vi "QCA.vi"() -> ()   [LabVIEW 2010]
uses:
  QCA Global.vi
panel:
  out "Sweep Done":refnum<k4>
  out "Mode Changed":refnum<k4>
  in  "stop":bool
  in  "Mode":T1(ring)
  out "QCA Message Type":T2(ring)=enum."MonitorDelay="
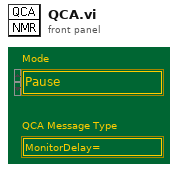
[diagram p1: front panel]
types:
  T1 = enum16{"Pause", "Take Data", "One Point", "NMR Tune", "Monitor"}
  T2 = enum16{"No Message", "Bad Message", "Init", "ChannelFile=", "RF On", "RF Off", "RFFreq=", "RFMod=", "RFPower=", "YaleGain=", "ScanSweeps=", "ScanSteps=", "ScanFreq=", "CalConst=", "MonitorDelay=", "Baseline=", "Baseline", "SaveChans", "Channel=", "Pause", "TakeData", "OnePoint", "NMRTune", "Monitor", "Address=", "Ping=", "Stop"}
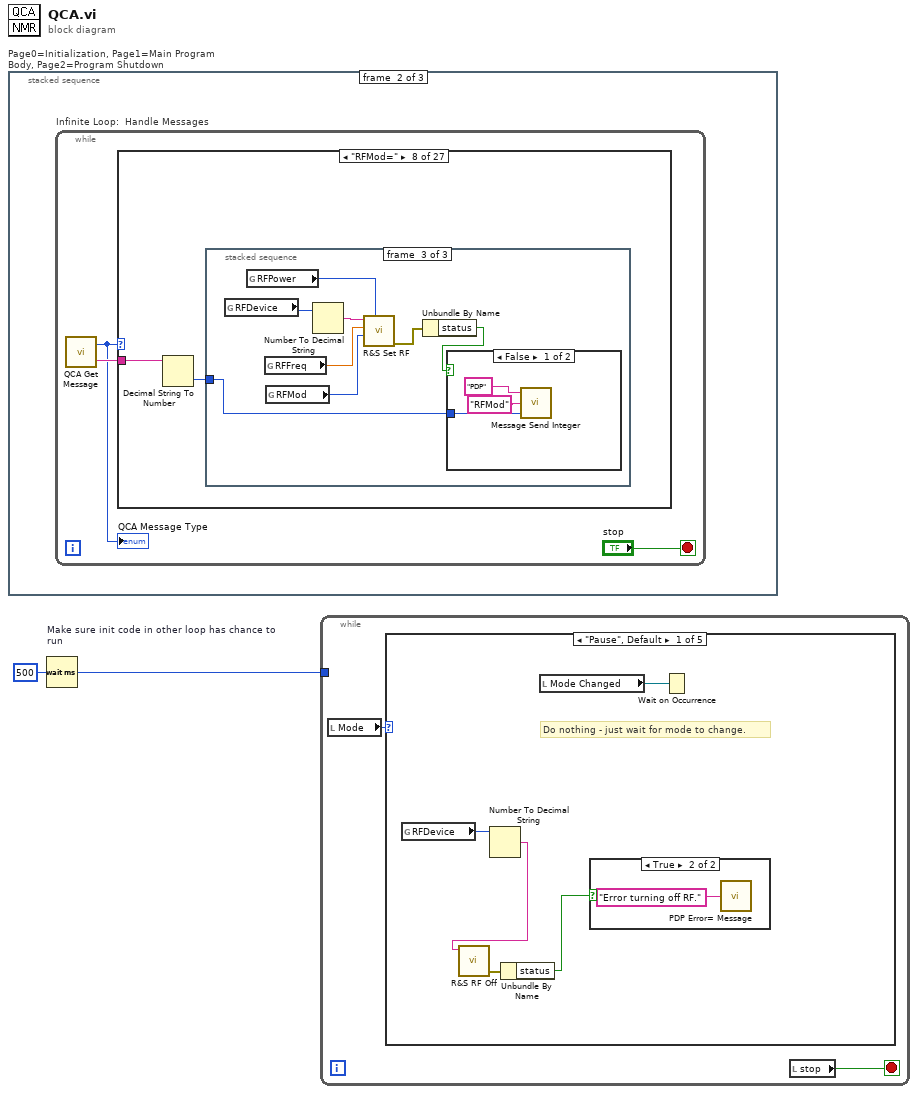
[diagram p0: block diagram]
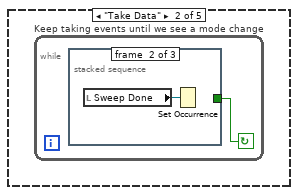
[diagram p3: hidden frame]
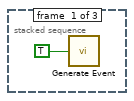
[diagram p4: hidden frame]
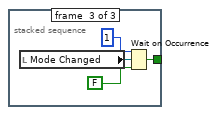
[diagram p5: hidden frame]
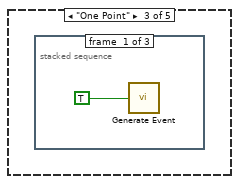
[diagram p6: hidden frame]
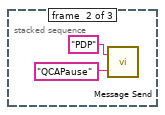
[diagram p7: hidden frame]
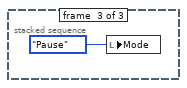
[diagram p8: hidden frame]
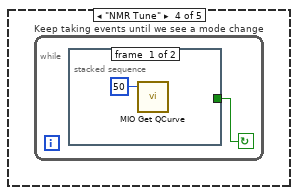
[diagram p9: hidden frame]
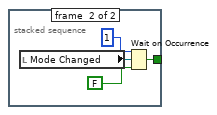
[diagram p10: hidden frame]
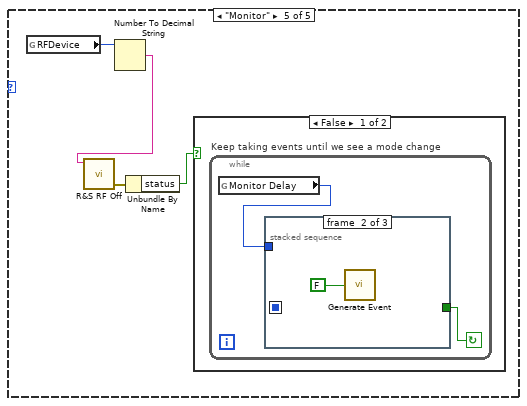
[diagram p11: hidden frame]
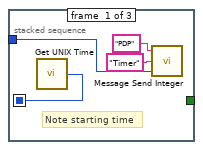
[diagram p12: hidden frame]
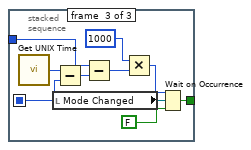
[diagram p13: hidden frame]
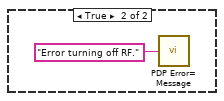
[diagram p14: hidden frame]
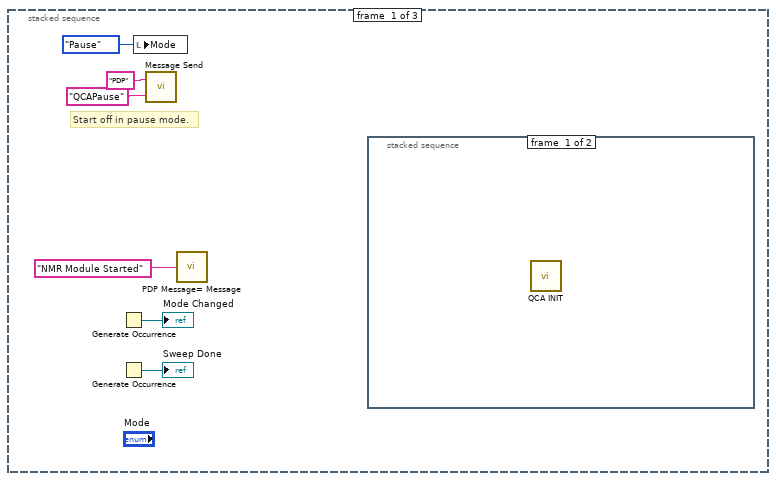
[diagram p15: hidden frame]
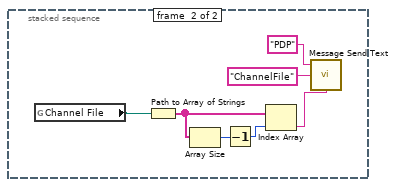
[diagram p16: hidden frame]
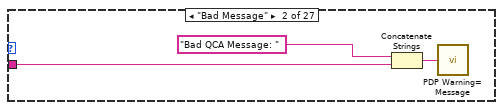
[diagram p18: hidden frame]
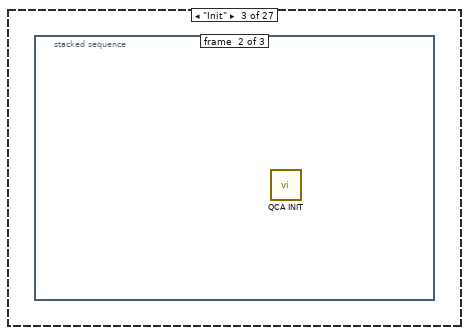
[diagram p19: hidden frame]
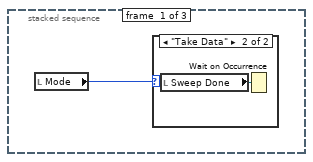
[diagram p20: hidden frame]
diagram:
  n1 = stacked-sequence "Page0=Initialization, Page1=Main Program Body, Page2=Program Shutdown" {
    frame #0 {
      # "Start off in pause mode."
      n2 = Generate Occurrence() -> (→"Mode Changed":refnum<k4>)
      n3 = Generate Occurrence() -> (→"Sweep Done":refnum<k4>)
      n4 = local write "Mode"(T1."Pause" ("Mode")) -> ()
      n5 = call "Message Send.vi"("Message"="QCAPause", "Destination"="PDP") -> ()
      n6 = call "PDP Message= Message.vi"("Message"="NMR Module Started") -> ()
      n7 = stacked-sequence {
        frame #0 {
          n8 = call "QCA INIT.vi"() -> ()  [unwired: 1 in]
        }
        frame #1 {
          n9 = global read "QCA Global.vi" "Channel File"() -> (w15:path)
          n10 = Path to Array of Strings(0:w15) -> (2:w11:string[])  [unwired: 1 out]
          n11 = Array Size(array=w11) -> (size(s)=w10:i32)
          n12 = Decrement(x=w10) -> (x-1=w9:i32)
          n13 = Index Array(array=w11, index=w9) -> (element=w12:string)
          n14 = call "Message Send Text.vi"("Value"=w12, "Parameter"="ChannelFile", "Destination"="PDP") -> ()
        }
      }
    }
    frame #1 {
      n15 = while "Infinite Loop:  Handle Messages" {
        stop <- "stop" stop-if-true
        n16 = call "QCA Get Message.vi"() -> ("QCA Message Type"=w17:T2, "Text"=w18:string)  [unwired: 1 in]
        "QCA Message Type" <- w17
        n17 = case shown="\"RFMod=\"" w17 {
          tunnel: w18 -> [_ w19 _ w25 _ _ w44 w61 w78 w95 w108 w110 w126 w130 w132 w134 _ _ w155 _ _ _ _ _ w216 w219 _]
          frame "No Message" {
          }
          frame "Bad Message" {
            n18 = Concatenate Strings("Bad QCA Message: ", w19) -> (w20:string)
            n19 = call "PDP Warning= Message.vi"("Message"=w20) -> ()
          }
          frame "Init" {
            n20 = stacked-sequence {
              frame #0 {
                n21 = local read "Mode"() -> (w22:T1)
                n22 = case shown="\"Take Data\"" w22 {
                  frame "Pause", Default {
                  }
                  frame "Take Data" {
                    n23 = local read "Sweep Done"() -> (w23:refnum<k4>)
                    n24 = Wait on Occurrence(2:w23) -> ()  [unwired: 2 in, 1 out]
                  }
                }
              }
              frame #1 {
                n25 = call "QCA INIT.vi"() -> ()  [unwired: 1 in]
              }
              frame #2 {
                n26 = call "PDP Message= Message.vi"("Message"="QCA Initialized") -> ()
              }
            }
          }
          frame "ChannelFile=" {
            n27 = stacked-sequence {
              tunnel: w25 -> [_ w31 _ _]
              frame #0 {
                n28 = local read "Mode"() -> (w26:T1)
                n29 = case shown="\"Take Data\"" w26 {
                  frame "Pause", Default {
                  }
                  frame "Take Data" {
                    n30 = local read "Sweep Done"() -> (w27:refnum<k4>)
                    n31 = Wait on Occurrence(2:w27) -> ()  [unwired: 2 in, 1 out]
                  }
                }
              }
              frame #1 {
                n32 = Build Array(w31) -> (w29:string[])
                n33 = Array of Strings to Path(0:w29, 1:TRUE ("relative")) -> (2:w30:path)
                n34 = global write "QCA Global.vi" "Channel File"(w30) -> ()
              }
              frame #2 {
                n35 = stacked-sequence "Read channels and set channel 0 as active." {
                  frame #0 {
                    n36 = global write "QCA Global.vi" "Current Channel"(-1 ("Current Channel")) -> ()
                  }
                  frame #1 {
                    n37 = call "QCA Init Channels.vi"() -> ()  [unwired: 1 in]
                  }
                  frame #2 {
                    n38 = call "QCA Get Channel Names.vi"() -> ("Channel Names"=w33:string[])
                    n39 = call "PDP Channels= Message.vi"("Channel"=w33) -> ()
                  }
                  frame #3 {
                    n40 = call "QCA Change Channels.vi"("Channel"=0) -> ()
                  }
                  frame #4 {
                    n41 = global read "QCA Global.vi" "Current Channel"() -> (w37:i32)
                    n42 = call "Message Send Integer.vi"("Value"=w37, "Parameter"="Channel", "Destination"="PDP") -> ()
                  }
                }
              }
              frame #3 {
                n43 = call "PDP Message= Message.vi"("Message"="Channel File Loaded") -> ()
              }
            }
          }
          frame "RF On" {
            n44 = global read "QCA Global.vi" "RFDevice"() -> (w40:i32)
            n45 = Number To Decimal String(number=w40) -> (decimal integer string=w39:string)  [unwired: 1 in]
            n46 = call "R&S RF On.vi"("address"=w39) -> ()  [unwired: 5 in, 2 out]
          }
          frame "RF Off" {
            n47 = global read "QCA Global.vi" "RFDevice"() -> (w42:i32)
            n48 = Number To Decimal String(number=w42) -> (decimal integer string=w41:string)  [unwired: 1 in]
            n49 = call "R&S RF Off.vi"("address"=w41) -> ()  [unwired: 5 in, 2 out]
          }
          frame "RFFreq=" {
            n50 = Fract/Exp String To Number(string=w44) -> (number=w43:dbl)  [unwired: 3 in, 1 out]
            n51 = stacked-sequence {
              tunnel: w43 -> [_ w47 w55]
              frame #0 {
                n52 = local read "Mode"() -> (w45:T1)
                n53 = case shown="\"Take Data\"" w45 {
                  frame "Pause", Default {
                  }
                  frame "Take Data" {
                    n54 = local read "Sweep Done"() -> (w46:refnum<k4>)
                    n55 = Wait on Occurrence(2:w46) -> ()  [unwired: 2 in, 1 out]
                  }
                }
              }
              frame #1 {
                n56 = global write "QCA Global.vi" "RFFreq"(w47) -> ()
              }
              frame #2 {
                n57 = global read "QCA Global.vi" "RFDevice"() -> (w50:i32)
                n58 = global read "QCA Global.vi" "RFPower"() -> (w52:i32)
                n59 = global read "QCA Global.vi" "RFFreq"() -> (w53:dbl)
                n60 = global read "QCA Global.vi" "RFMod"() -> (w54:i32)
                n61 = Number To Decimal String(number=w50) -> (decimal integer string=w51:string)  [unwired: 1 in]
                n62 = call "R&S Set RF.vi"("power (mW)"=w52, "modulation (kHz)"=w54, "center frequency (Hz)"=w53, "address"=w51) -> ("error out"=w49:errorcluster)  [unwired: 3 in, 1 out]
                n63 = Unbundle By Name(w49) -> ("status"=w48:bool)
                n64 = case shown="False" w48 {
                  tunnel: w55 -> [w56 _]
                  frame False {
                    n65 = call "Message Send Float.vi"("Value"=w56, "Parameter"="RFFreq", "Destination"="PDP") -> ()
                  }
                  frame True {
                    n66 = call "PDP Error= Message.vi"("Message"="Error=Error Setting RF Frequency.") -> ()
                  }
                }
              }
            }
          }
          frame "RFMod=" {
            n67 = Decimal String To Number(string=w61) -> (number=w60:i32)  [unwired: 2 in, 1 out]
            n68 = stacked-sequence {
              tunnel: w60 -> [_ w64 w72]
              frame #0 {
                n69 = local read "Mode"() -> (w62:T1)
                n70 = case shown="\"Take Data\"" w62 {
                  frame "Pause", Default {
                  }
                  frame "Take Data" {
                    n71 = local read "Sweep Done"() -> (w63:refnum<k4>)
                    n72 = Wait on Occurrence(2:w63) -> ()  [unwired: 2 in, 1 out]
                  }
                }
              }
              frame #1 {
                n73 = global write "QCA Global.vi" "RFMod"(w64) -> ()
              }
              frame #2 {
                n74 = global read "QCA Global.vi" "RFDevice"() -> (w67:i32)
                n75 = global read "QCA Global.vi" "RFPower"() -> (w69:i32)
                n76 = global read "QCA Global.vi" "RFFreq"() -> (w70:dbl)
                n77 = global read "QCA Global.vi" "RFMod"() -> (w71:i32)
                n78 = Number To Decimal String(number=w67) -> (decimal integer string=w68:string)  [unwired: 1 in]
                n79 = call "R&S Set RF.vi"("power (mW)"=w69, "modulation (kHz)"=w71, "center frequency (Hz)"=w70, "address"=w68) -> ("error out"=w66:errorcluster)  [unwired: 3 in, 1 out]
                n80 = Unbundle By Name(w66) -> ("status"=w65:bool)
                n81 = case shown="False" w65 {
                  tunnel: w72 -> [w75 _]
                  frame False {
                    n82 = call "Message Send Integer.vi"("Value"=w75, "Parameter"="RFMod", "Destination"="PDP") -> ()
                  }
                  frame True {
                    n83 = call "PDP Error= Message.vi"("Message"="Error=Error Setting RF Modulation.") -> ()
                  }
                }
              }
            }
          }
          frame "RFPower=" {
            n84 = Decimal String To Number(string=w78) -> (number=w77:i32)  [unwired: 2 in, 1 out]
            n85 = stacked-sequence {
              tunnel: w77 -> [_ w81 w89]
              frame #0 {
                n86 = local read "Mode"() -> (w79:T1)
                n87 = case shown="\"Take Data\"" w79 {
                  frame "Pause", Default {
                  }
                  frame "Take Data" {
                    n88 = local read "Sweep Done"() -> (w80:refnum<k4>)
                    n89 = Wait on Occurrence(2:w80) -> ()  [unwired: 2 in, 1 out]
                  }
                }
              }
              frame #1 {
                n90 = global write "QCA Global.vi" "RFPower"(w81) -> ()
              }
              frame #2 {
                n91 = global read "QCA Global.vi" "RFDevice"() -> (w84:i32)
                n92 = global read "QCA Global.vi" "RFPower"() -> (w86:i32)
                n93 = global read "QCA Global.vi" "RFFreq"() -> (w87:dbl)
                n94 = global read "QCA Global.vi" "RFMod"() -> (w88:i32)
                n95 = Number To Decimal String(number=w84) -> (decimal integer string=w85:string)  [unwired: 1 in]
                n96 = call "R&S Set RF.vi"("power (mW)"=w86, "modulation (kHz)"=w88, "center frequency (Hz)"=w87, "address"=w85) -> ("error out"=w83:errorcluster)  [unwired: 3 in, 1 out]
                n97 = Unbundle By Name(w83) -> ("status"=w82:bool)
                n98 = case shown="False" w82 {
                  tunnel: w89 -> [w92 _]
                  frame False {
                    n99 = call "Message Send Integer.vi"("Value"=w92, "Parameter"="RFPower", "Destination"="PDP") -> ()
                  }
                  frame True {
                    n100 = call "PDP Error= Message.vi"("Message"="Error=Error Setting RF Power.") -> ()
                  }
                }
              }
            }
          }
          frame "YaleGain=" {
            n101 = Decimal String To Number(string=w95) -> (number=w94:i32)  [unwired: 2 in, 1 out]
            n102 = stacked-sequence {
              tunnel: w94 -> [_ w98 w99]
              frame #0 {
                n103 = local read "Mode"() -> (w96:T1)
                n104 = case shown="\"Take Data\"" w96 {
                  frame "Pause", Default {
                  }
                  frame "Take Data" {
                    n105 = local read "Sweep Done"() -> (w97:refnum<k4>)
                    n106 = Wait on Occurrence(2:w97) -> ()  [unwired: 2 in, 1 out]
                  }
                }
              }
              frame #1 {
                n107 = global write "QCA Global.vi" "YaleGain"(w98) -> ()
              }
              frame #2 {
                n108 = call "Yale Set Gain.vi"() -> ("Error"=w100:bool)
                n109 = case shown="False" w100 {
                  tunnel: w99 -> [w103 _]
                  frame False {
                    n110 = call "Message Send Integer.vi"("Value"=w103, "Parameter"="YaleGain", "Destination"="PDP") -> ()
                  }
                  frame True {
                    n111 = call "PDP Error= Message.vi"("Message"="Error=Error Setting Yale Gain.") -> ()
                  }
                }
              }
            }
          }
          frame "ScanSweeps=" {
            n112 = Decimal String To Number(string=w108) -> (number=w107:i32)  [unwired: 2 in, 1 out]
            n113 = global write "QCA Global.vi" "ScanSweeps"(w107) -> ()
            n114 = call "Message Send Integer.vi"("Value"=w107, "Parameter"="ScanSweeps", "Destination"="PDP") -> ()
          }
          frame "ScanSteps=" {
            n115 = Decimal String To Number(string=w110) -> (number=w109:i32)  [unwired: 2 in, 1 out]
            n116 = stacked-sequence {
              tunnel: w109 -> [w111 w115 w122]
              frame #0 {
                n117 = global write "QCA Global.vi" "ScanSteps"(w111) -> ()
              }
              frame #1 {
                # "setup ramp"
                n118 = for {
                  N: w115 -> [_]
                  tunnel: [w119] -> w118 mode=indexing
                  i -> [w119]
                }
                n119 = Compound Arithmetic op=MULTIPLY(w118, invert w115, 2 ("Input")) -> (w116:dbl[])
                n120 = Decrement(x=w116) -> (x-1=w113:dbl[])
                n121 = Reverse 1D Array(array=w113) -> (reversed array=w114:dbl[])
                n122 = Build Array (concatenate)(w113, w114) -> (w112:dbl[])
                n123 = global write "QCA Global.vi" "ScanRamp"(w112) -> ()
              }
              frame #2 {
                n124 = call "Message Send Integer.vi"("Value"=w122, "Parameter"="ScanSteps", "Destination"="PDP") -> ()
              }
            }
          }
          frame "ScanFreq=" {
            n125 = Decimal String To Number(string=w126) -> (number=w125:i32)  [unwired: 2 in, 1 out]
            n126 = global write "QCA Global.vi" "ScanFreq"(w125) -> ()
            n127 = call "Message Send Integer.vi"("Value"=w125, "Parameter"="ScanFreq", "Destination"="PDP") -> ()
          }
          frame "CalConst=" {
            n128 = Fract/Exp String To Number(string=w130) -> (number=w129:dbl)  [unwired: 3 in, 1 out]
            n129 = global write "QCA Global.vi" "CalConst"(w129) -> ()
            n130 = call "Message Send Float.vi"("Value"=w129, "Parameter"="CalConst", "Destination"="PDP") -> ()
          }
          frame "MonitorDelay=" {
            n131 = Decimal String To Number(string=w132) -> (number=w131:i32)  [unwired: 2 in, 1 out]
            n132 = global write "QCA Global.vi" "Monitor Delay"(w131) -> ()
          }
          frame "Baseline=" {
            n133 = Decimal String To Number(string=w134) -> (number=w133:i32)  [unwired: 2 in, 1 out]
            n134 = global write "QCA Global.vi" "Baseline"(w133) -> ()
            n135 = case shown="1, Default" w133 {
              tunnel: w133 -> [_ _ w141]
              tunnel: ["New Baseline" ("TimeStamp") "No Baseline" ("TimeStamp") w140] -> w135
              frame 0 {
              }
              frame -1 {
              }
              frame 1, Default {
                n136 = call "Event Number to Timestamp.vi"("Event Number"=w141) -> ("TimeStamp"=w140:string)
              }
            }
            n137 = call "Message Send Text.vi"("Value"=w135, "Parameter"="Baseline", "Destination"="PDP") -> ()
          }
          frame "Baseline" {
            n138 = global read "QCA Global.vi" "QMeterName"() -> (w146:string)
            n139 = global read "QCA Global.vi" "Baseline"() -> (w147:i32)
            n140 = call "QCA Pick Baseline.vi"("QMeter"=w146, "Current Baseline"=w147) -> ("New Baseline"=w142:i32)
            n141 = global write "QCA Global.vi" "Baseline"(w142) -> ()
            n142 = case shown="1, Default" w142 {
              tunnel: w142 -> [_ _ w151]
              tunnel: ["New Baseline" ("TimeStamp") "No Baseline" ("TimeStamp") w150] -> w143
              frame 0 {
              }
              frame -1 {
              }
              frame 1, Default {
                n143 = call "Event Number to Timestamp.vi"("Event Number"=w151) -> ("TimeStamp"=w150:string)
              }
            }
            n144 = call "Message Send Text.vi"("Value"=w143, "Parameter"="Baseline", "Destination"="PDP") -> ()
          }
          frame "SaveChans" {
            n145 = call "QCA Save Channels.vi"() -> ("Error"=w152:bool)
            n146 = case shown="False" w152 {
              frame False {
                n147 = call "PDP Message= Message.vi"("Message"="Channels Saved.") -> ()
              }
              frame True {
                n148 = call "PDP Error= Message.vi"("Message"="Error saving channels.") -> ()
              }
            }
          }
          frame "Channel=" {
            n149 = stacked-sequence {
              tunnel: w155 -> [_ w159]
              frame #0 {
                n150 = local read "Mode"() -> (w156:T1)
                n151 = case shown="\"Take Data\"" w156 {
                  frame "Pause", Default {
                  }
                  frame "Take Data" {
                    n152 = local read "Sweep Done"() -> (w157:refnum<k4>)
                    n153 = Wait on Occurrence(2:w157) -> ()  [unwired: 2 in, 1 out]
                  }
                }
              }
              frame #1 {
                n154 = Decimal String To Number(string=w159) -> (number=w158:i32)  [unwired: 2 in, 1 out]
                n155 = call "QCA Change Channels.vi"("Channel"=w158) -> ()
              }
            }
          }
          frame "Pause" {
            n156 = stacked-sequence {
              frame #0 {
                n157 = local read "Mode"() -> (w160:T1)
                n158 = case shown="\"Take Data\"" w160 {
                  frame "Pause", Default {
                  }
                  frame "Take Data" {
                    n159 = local read "Sweep Done"() -> (w161:refnum<k4>)
                    n160 = Wait on Occurrence(2:w161) -> ()  [unwired: 2 in, 1 out]
                  }
                }
              }
              frame #1 {
                n161 = local write "Mode"(T1."Pause" ("Mode")) -> ()
              }
              frame #2 {
                n162 = local read "Mode Changed"() -> (w163:refnum<k4>)
                n163 = Set Occurrence(w163) -> ()
              }
              frame #3 {
                n164 = call "Message Send.vi"("Message"="QCAPause", "Destination"="PDP") -> ()
              }
            }
          }
          frame "TakeData" {
            n165 = global read "QCA Global.vi" "RFDevice"() -> (w167:i32)
            n166 = Number To Decimal String(number=w167) -> (decimal integer string=w166:string)  [unwired: 1 in]
            n167 = call "R&S RF On.vi"("address"=w166) -> ("error out"=w169:errorcluster)  [unwired: 5 in, 1 out]
            n168 = Unbundle By Name(w169) -> ("status"=w168:bool)
            n169 = case shown="True" w168 {
              frame False {
                n170 = stacked-sequence {
                  frame #0 {
                    n171 = local write "Mode"(T1."Take Data" ("Mode")) -> ()
                  }
                  frame #1 {
                    n172 = local read "Mode Changed"() -> (w171:refnum<k4>)
                    n173 = Set Occurrence(w171) -> ()
                  }
                  frame #2 {
                    n174 = call "Message Send.vi"("Message"="QCATakeData", "Destination"="PDP") -> ()
                  }
                }
              }
              frame True {
                n175 = stacked-sequence {
                  frame #0 {
                    n176 = local write "Mode"(T1."Pause" ("Mode")) -> ()
                  }
                  frame #1 {
                    n177 = local read "Mode Changed"() -> (w175:refnum<k4>)
                    n178 = Set Occurrence(w175) -> ()
                  }
                  frame #2 {
                    n179 = call "Message Send.vi"("Message"="QCAPause", "Destination"="PDP") -> ()
                  }
                  frame #3 {
                    n180 = call "PDP Error= Message.vi"("Message"="Error turning on RF.") -> ()
                  }
                }
              }
            }
          }
          frame "OnePoint" {
            n181 = global read "QCA Global.vi" "RFDevice"() -> (w182:i32)
            n182 = Number To Decimal String(number=w182) -> (decimal integer string=w181:string)  [unwired: 1 in]
            n183 = call "R&S RF On.vi"("address"=w181) -> ("error out"=w180:errorcluster)  [unwired: 5 in, 1 out]
            n184 = Unbundle By Name(w180) -> ("status"=w179:bool)
            n185 = case shown="False" w179 {
              frame False {
                n186 = stacked-sequence {
                  frame #0 {
                    n187 = local write "Mode"(T1."One Point" ("Mode")) -> ()
                  }
                  frame #1 {
                    n188 = local read "Mode Changed"() -> (w184:refnum<k4>)
                    n189 = Set Occurrence(w184) -> ()
                  }
                  frame #2 {
                    n190 = call "Message Send.vi"("Message"="QCATakeData", "Destination"="PDP") -> ()
                  }
                }
              }
              frame True {
                n191 = stacked-sequence {
                  frame #0 {
                    n192 = local write "Mode"(T1."Pause" ("Mode")) -> ()
                  }
                  frame #1 {
                    n193 = local read "Mode Changed"() -> (w188:refnum<k4>)
                    n194 = Set Occurrence(w188) -> ()
                  }
                  frame #2 {
                    n195 = call "Message Send.vi"("Message"="QCAPause", "Destination"="PDP") -> ()
                  }
                  frame #3 {
                    n196 = call "PDP Error= Message.vi"("Message"="Error turning on RF.") -> ()
                  }
                }
              }
            }
          }
          frame "NMRTune" {
            n197 = stacked-sequence {
              frame #0 {
                n198 = local read "Mode"() -> (w192:T1)
                n199 = case shown="\"Take Data\"" w192 {
                  frame "Pause", Default {
                  }
                  frame "Take Data" {
                    n200 = local read "Sweep Done"() -> (w193:refnum<k4>)
                    n201 = Wait on Occurrence(2:w193) -> ()  [unwired: 2 in, 1 out]
                  }
                }
              }
              frame #1 {
                n202 = global read "QCA Global.vi" "RFDevice"() -> (w197:i32)
                n203 = Number To Decimal String(number=w197) -> (decimal integer string=w196:string)  [unwired: 1 in]
                n204 = call "R&S RF On.vi"("address"=w196) -> ("error out"=w195:errorcluster)  [unwired: 5 in, 1 out]
                n205 = Unbundle By Name(w195) -> ("status"=w194:bool)
                n206 = case shown="False" w194 {
                  frame False {
                    n207 = stacked-sequence {
                      frame #0 {
                        n208 = local write "Mode"(T1."NMR Tune" ("Mode")) -> ()
                      }
                      frame #1 {
                        n209 = local read "Mode Changed"() -> (w199:refnum<k4>)
                        n210 = Set Occurrence(w199) -> ()
                      }
                      frame #2 {
                        n211 = call "Message Send.vi"("Message"="QCANMRTune", "Destination"="PDP") -> ()
                      }
                    }
                  }
                  frame True {
                    n212 = stacked-sequence {
                      frame #0 {
                        n213 = local write "Mode"(T1."Pause" ("Mode")) -> ()
                      }
                      frame #1 {
                        n214 = local read "Mode Changed"() -> (w203:refnum<k4>)
                        n215 = Set Occurrence(w203) -> ()
                      }
                      frame #2 {
                        n216 = call "Message Send.vi"("Message"="QCAPause", "Destination"="PDP") -> ()
                      }
                      frame #3 {
                        n217 = call "PDP Error= Message.vi"("Message"="Error turning on RF.") -> ()
                      }
                    }
                  }
                }
              }
            }
          }
          frame "Monitor" {
            n218 = stacked-sequence {
              frame #0 {
                n219 = local read "Mode"() -> (w207:T1)
                n220 = case shown="\"Take Data\"" w207 {
                  frame "Pause", Default {
                  }
                  frame "Take Data" {
                    n221 = local read "Sweep Done"() -> (w208:refnum<k4>)
                    n222 = Wait on Occurrence(2:w208) -> ()  [unwired: 2 in, 1 out]
                  }
                }
              }
              frame #1 {
                n223 = local write "Mode"(T1."Monitor" ("Mode")) -> ()
              }
              frame #2 {
                n224 = local read "Mode Changed"() -> (w210:refnum<k4>)
                n225 = Set Occurrence(w210) -> ()
              }
              frame #3 {
                n226 = call "Message Send.vi"("Message"="QCAMonitor", "Destination"="PDP") -> ()
              }
            }
          }
          frame "Address=" {
            n227 = Scan From String(format string="%s,%[.0-9]:%d" ("Format String"), input string=w216) -> (output 1=w214:string, output 2=w215:string, output 3=w213:i32)  [unwired: 5 in, 3 out]
            n228 = call "Message Set Module Address.vi"("Port"=w213, "Address"=w215, "Module"=w214) -> ()
          }
          frame "Ping=" {
            n229 = Get Date/Time In Seconds() -> (seconds since 1Jan1904=w218:timestamp)
            n230 = To Double Precision Float(number=w218) -> (double precision float=w221:dbl)
            n231 = Format Into String(format string="PingResponse=QCA,%.0f", w221) -> (resulting string=w220:string)  [unwired: 2 in, 1 out]
            n232 = call "Message Send.vi"("Message"=w220, "Destination"=w219) -> ()
          }
          frame "Stop" {
            n233 = local write "stop"(TRUE ("stop")) -> ()
          }
        }
      }
    }
    frame #2 {
      n234 = call "PDP Message= Message.vi"("Message"="QCA Module Stopped") -> ()
    }
  }
  n235 = Wait (ms) "Make sure init code in other loop has chance to run"(milliseconds to wait=u32 500) -> (millisecond timer value=w1:u32)
  n236 = while {
    tunnel: w1 -> [_]
    stop <- w225 stop-if-true
    n237 = local read "Mode"() -> (w226:T1)
    n238 = case shown="\"Pause\", Default" w226 {
      frame "Pause", Default {
        # "Do nothing - just wait for mode to change."
        n239 = global read "QCA Global.vi" "RFDevice"() -> (w230:i32)
        n240 = Number To Decimal String(number=w230) -> (decimal integer string=w229:string)  [unwired: 1 in]
        n241 = call "R&S RF Off.vi"("address"=w229) -> ("error out"=w228:errorcluster)  [unwired: 5 in, 1 out]
        n242 = Unbundle By Name(w228) -> ("status"=w227:bool)
        n243 = local read "Mode Changed"() -> (w231:refnum<k4>)
        n244 = case shown="True" w227 {
          frame False {
          }
          frame True {
            n245 = call "PDP Error= Message.vi"("Message"="Error turning off RF.") -> ()
          }
        }
        n246 = Wait on Occurrence(2:w231) -> ()  [unwired: 2 in, 1 out]
      }
      frame "Take Data" {
        n247 = while "Keep taking events until we see a mode change" {
          stop <- w233 continue-if-true
          n248 = stacked-sequence {
            tunnel: [_ _ w239] -> w233
            frame #0 {
              n249 = call "Generate Event.vi"("Include NMR Data"=TRUE) -> ()
            }
            frame #1 {
              n250 = local read "Sweep Done"() -> (w235:refnum<k4>)
              n251 = Set Occurrence(w235) -> ()
            }
            frame #2 {
              n252 = local read "Mode Changed"() -> (w238:refnum<k4>)
              n253 = Wait on Occurrence(1:FALSE ("ignore previous (T)"), 2:w238, 3:1 ("ms timeout (-1)")) -> (0:w239:bool)
            }
          }
        }
      }
      frame "One Point" {
        n254 = stacked-sequence {
          frame #0 {
            n255 = call "Generate Event.vi"("Include NMR Data"=TRUE) -> ()
          }
          frame #1 {
            n256 = call "Message Send.vi"("Message"="QCAPause", "Destination"="PDP") -> ()
          }
          frame #2 {
            n257 = local write "Mode"(T1."Pause" ("Mode")) -> ()
          }
        }
      }
      frame "NMR Tune" {
        n258 = while "Keep taking events until we see a mode change" {
          stop <- w244 continue-if-true
          n259 = stacked-sequence {
            tunnel: [_ w249] -> w244
            frame #0 {
              n260 = call "MIO Get QCurve.vi"("Num Sweeps"=50) -> ()  [unwired: 2 in, 1 out]
            }
            frame #1 {
              n261 = local read "Mode Changed"() -> (w248:refnum<k4>)
              n262 = Wait on Occurrence(1:FALSE ("ignore previous (T)"), 2:w248, 3:1 ("ms timeout (-1)")) -> (0:w249:bool)
            }
          }
        }
      }
      frame "Monitor" {
        n263 = global read "QCA Global.vi" "RFDevice"() -> (w253:i32)
        n264 = Number To Decimal String(number=w253) -> (decimal integer string=w252:string)  [unwired: 1 in]
        n265 = call "R&S RF Off.vi"("address"=w252) -> ("error out"=w251:errorcluster)  [unwired: 5 in, 1 out]
        n266 = Unbundle By Name(w251) -> ("status"=w250:bool)
        n267 = case shown="False" w250 {
          frame False {
            n268 = while "Keep taking events until we see a mode change" {
              stop <- w255 continue-if-true
              n269 = global read "QCA Global.vi" "Monitor Delay"() -> (w254:i32)
              n270 = stacked-sequence {
                seq-local: [w259 _ _] -> [_ _ w268]
                tunnel: [_ _ w270] -> w255
                tunnel: w254 -> [w256 _ w262]
                frame #0 {
                  # "Note starting time"
                  n271 = call "Get UNIX Time.vi"() -> ("UNIX seconds"=w259:i32)
                  n272 = call "Message Send Integer.vi"("Value"=w256, "Parameter"="Timer", "Destination"="PDP") -> ()
                }
                frame #1 {
                  n273 = call "Generate Event.vi"("Include NMR Data"=FALSE) -> ()
                }
                frame #2 {
                  n274 = call "Get UNIX Time.vi"() -> ("UNIX seconds"=w267:i32)
                  n275 = local read "Mode Changed"() -> (w269:refnum<k4>)
                  n276 = Subtract(x=w267, y=w268) -> (x-y=w266:i32)
                  n277 = Subtract(x=w262, y=w266) -> (x-y=w265:i32)
                  n278 = Multiply(x=1000, y=w265) -> (x*y=w263:i32)
                  n279 = Wait on Occurrence(1:FALSE ("ignore previous (T)"), 2:w269, 3:w263) -> (0:w270:bool)
                }
              }
            }
          }
          frame True {
            n280 = call "PDP Error= Message.vi"("Message"="Error turning off RF.") -> ()
          }
        }
      }
    }
    n281 = local read "stop"() -> (w225:bool)
  }
